vi "Valid AutoPopulate.vi"(0 "Starting Serial Number":u32, 7 "Ending Serial Number":u32, 11 "Serial Number Step":u32) -> (8 "Valid?":bool)   [LabVIEW 2013]
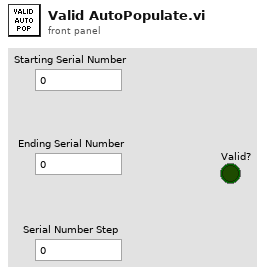
[diagram p1: front panel]
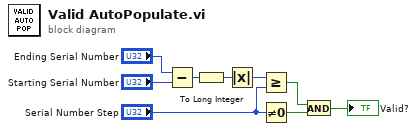
[diagram p0: block diagram]
diagram:
  n1 = Subtract(x="Ending Serial Number", y="Starting Serial Number") -> (x-y=w5:u32)
  n2 = To Long Integer(number=w5) -> (32bit integer=w6:i32)
  n3 = Absolute Value(x=w6) -> (abs(x)=w7:i32)
  n4 = Greater Or Equal?(x=w7, y="Serial Number Step") -> (x >= y?=w9:bool)
  n5 = Not Equal To 0?(x="Serial Number Step") -> (x != 0?=w2:bool)
  n6 = And(x=w9, y=w2) -> (x .and. y?=→"Valid?":bool)
